vi "Front_ end_testcse.vi"() -> ()   [LabVIEW 2016]
uses:
  <vilib>/regexp/Match Regular Expression.xnode
  <vilib>/httpClient/LabVIEWHTTPClient.lvlib
panel:
  out "String":string
  out "?":dbl
  out "Number of Faulty Traffic LIghts":i32(knob) scale=0.0..34.0
  out "Faulty Signals":string[](array[string])
  out "List of Traffic  Signals":string[](array[string])
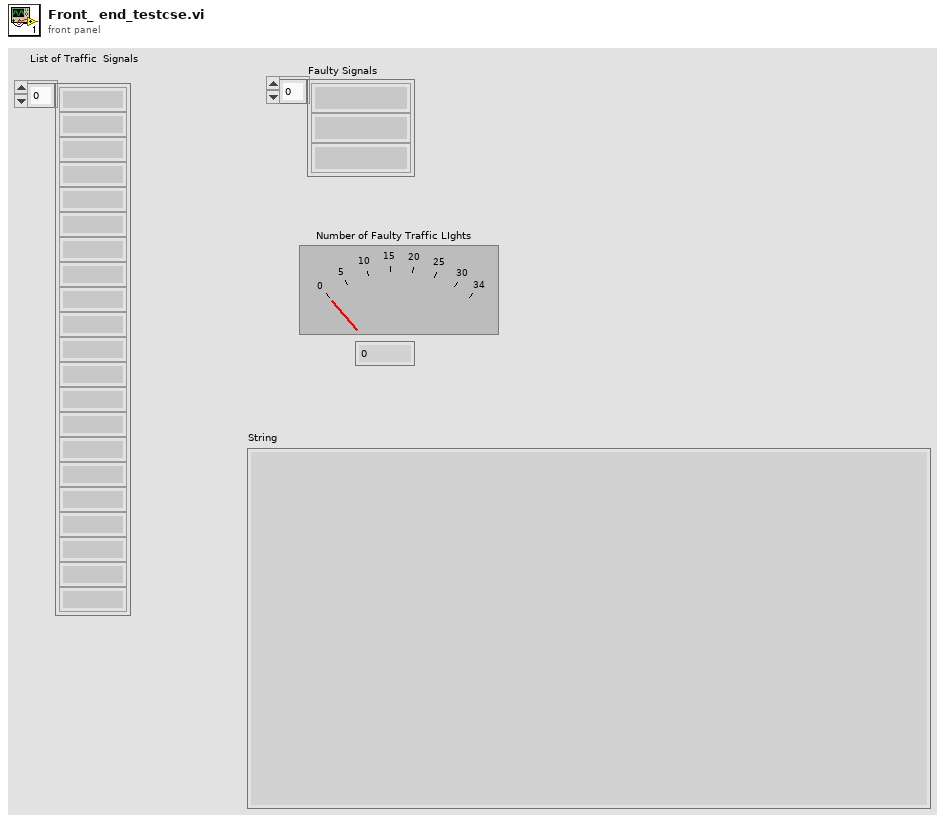
[diagram p1: front panel]
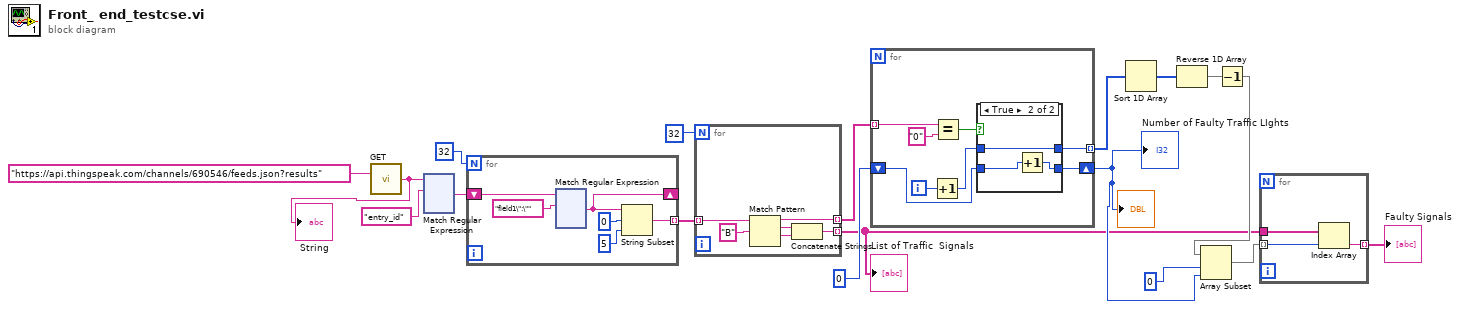
[diagram p0: block diagram]
diagram:
  n1 = call <vilib>:"GET.vi"("url"="https://api.thingspeak.com/channels/690546/feeds.json?results") -> ("body"=w1:string)  [unwired: 11 in, 3 out]
  "String" <- w1
  n2 = xnode "Match Regular Expression"("input string"=w1, "regular expression"="entry_id") -> ("after match"=w17:string)  [unwired: 4 in, 4 out]
  n3 = for {
    N: 32 -> [_]
    tunnel: [w21] -> w16 mode=indexing
    shift-right: [w19] -> _
    shift-left: w17 -> [w20]
    n4 = xnode "Match Regular Expression"("input string"=w20, "regular expression"="field1\":\"") -> ("after match"=w19:string)  [unwired: 4 in, 4 out]
    n5 = String Subset(string=w19, offset (0)=0, length (rest)=5) -> (substring=w21:string)
  }
  n6 = for {
    N: 32 -> [_]
    tunnel: w16 -> [w144] mode=indexing
    tunnel: [w142] -> w3 mode=indexing
    tunnel: [w139] -> w2 mode=indexing
    n7 = Match Pattern(string=w144, regular expression="B") -> (before substring=w142:string, match substring=w141:string, after substring=w140:string)  [unwired: 1 in, 1 out]
    n8 = Concatenate Strings(w141, w140) -> (w139:string)
  }
  "List of Traffic  Signals" <- w2
  n9 = for {
    tunnel: w3 -> [w152] mode=indexing
    tunnel: [w147] -> w12 mode=indexing
    shift-right: [w145] -> w5
    shift-left: 0 -> [w146]
    i -> [w149]
    n10 = Increment(x=w149) -> (x+1=w148:i32)
    n11 = Equal?(x=w152, y="0") -> (x = y?=w150:bool)
    n12 = case shown="True" w150 {
      tunnel: w148 -> [_ w156]
      tunnel: [_ w156] -> w147
      tunnel: w146 -> [w153 w155]
      tunnel: [w153 w154] -> w145
      frame False {
      }
      frame True {
        n13 = Increment(x=w155) -> (x+1=w154:i32)
      }
    }
  }
  "Number of Faulty Traffic LIghts" <- w5
  "?" <- w5
  n14 = Sort 1D Array(array=w12) -> (sorted array=w11:i32[])
  n15 = Reverse 1D Array(array=w11) -> (reversed array=w10:i32[])
  n16 = Decrement(x=w10) -> (x-1=w7:i32[])
  n17 = Array Subset(array=w7, index=0, length=w5) -> (w4:i32[])
  n18 = for {
    tunnel: [w159] -> w9 mode=indexing
    tunnel: w2 -> [w158]
    tunnel: w4 -> [w157] mode=indexing
    n19 = Index Array(array=w158, index=w157) -> (element=w159:string)
  }
  "Faulty Signals" <- w9
